vi "FuzzyMapToInt16.vi"(8 "Table Control":string[][](table)) -> (0 "Array 2":u16[](array[numeric]))   [LabVIEW 2016]
panel:
  out "Array":i32[](array[numeric])
  out "array":string[](array[string])
  out "output array":string[](array[string])
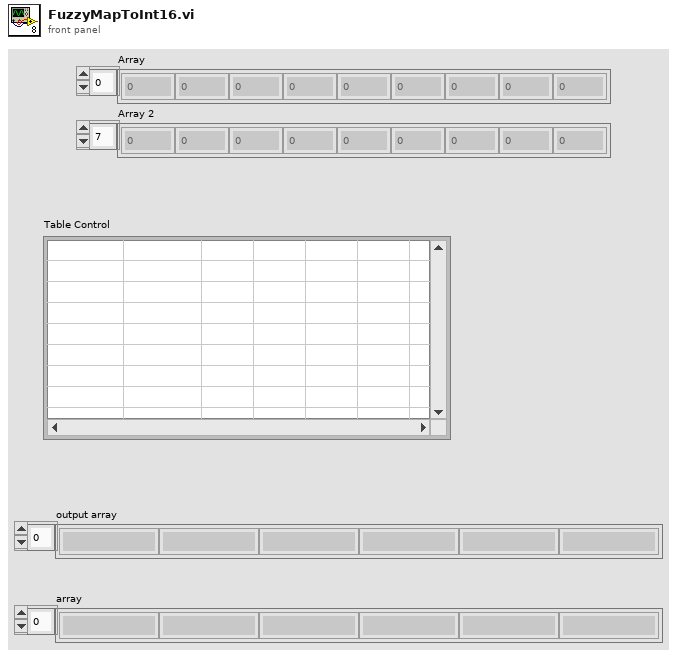
[diagram p1: front panel]
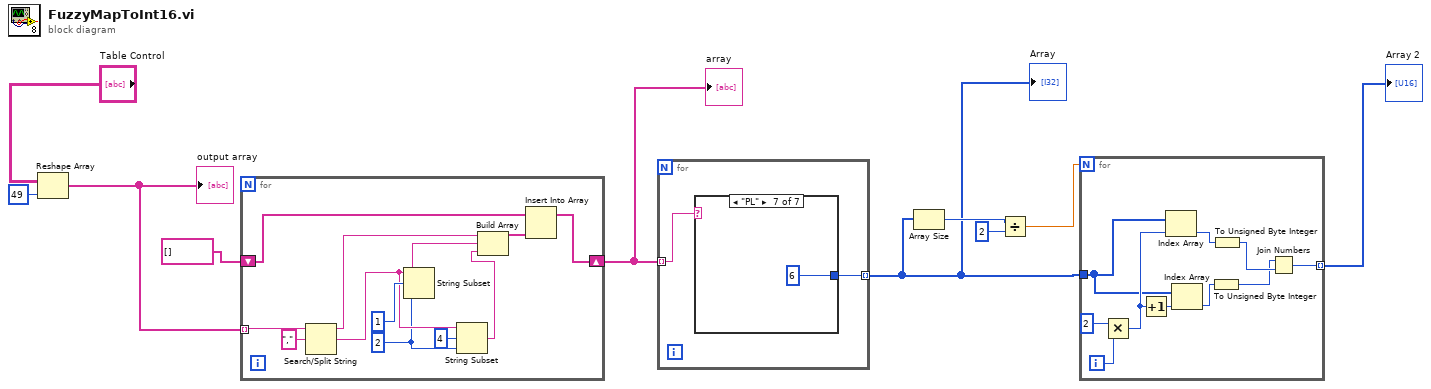
[diagram p0: block diagram]
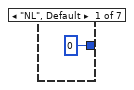
[diagram p2: hidden frame]
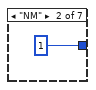
[diagram p3: hidden frame]
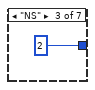
[diagram p4: hidden frame]
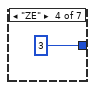
[diagram p5: hidden frame]
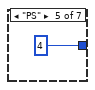
[diagram p6: hidden frame]
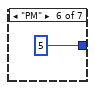
[diagram p7: hidden frame]
diagram:
  n1 = Reshape Array("Table Control", 49 ("dimension size")) -> (w8:string[])
  "output array" <- w8
  n2 = for {
    tunnel: w8 -> [w22] mode=indexing
    shift-right: [w17] -> w6
    shift-left: string[] [] ("array") -> [w18]
    w13 = 2 ("length (rest)")
    n3 = Search/Split String(string=w22, search string/char (-)=",") -> (substring before match=w20:string, match + rest of string=w14:string)  [unwired: 1 in, 1 out]
    n4 = String Subset(string=w14, offset (0)=1, length (rest)=w13) -> (substring=w15:string)
    n5 = String Subset(string=w14, offset (0)=4, length (rest)=w13) -> (substring=w11:string)
    n6 = Build Array(w20, w15, w11) -> (w19:string[])
    n7 = Insert Into Array(array=w18, new element=w19) -> (w17:string[])  [unwired: 1 in]
  }
  "array" <- w6
  n8 = for {
    tunnel: w6 -> [w24] mode=indexing
    tunnel: [w23] -> w2 mode=indexing
    n9 = case shown="\"PL\"" w24 {
      tunnel: [0 ("length (rest)") 1 ("length (rest)") 2 ("length (rest)") 3 ("length (rest)") 4 ("length (rest)") 5 ("length (rest)") 6 ("length (rest)")] -> w23
      frame "NL", Default {
      }
      frame "NM" {
      }
      frame "NS" {
      }
      frame "ZE" {
      }
      frame "PS" {
      }
      frame "PM" {
      }
      frame "PL" {
      }
    }
  }
  "Array" <- w2
  n10 = Array Size(array=w2) -> (size(s)=w5:i32)
  n11 = Divide(x=w5, y=2) -> (x/y=w3:dbl)
  n12 = for {
    N: w3 -> [_]
    tunnel: w2 -> [w37]
    tunnel: [w34] -> w1 mode=indexing
    i -> [w41]
    n13 = Multiply(x=2, y=w41) -> (x*y=w39:i32)
    n14 = Increment(x=w39) -> (x+1=w38:i32)
    n15 = Index Array(array=w37, index=w39) -> (element=w36:i32)
    n16 = Index Array(array=w37, index=w38) -> (element=w35:i32)
    n17 = To Unsigned Byte Integer(number=w35) -> (unsigned 8bit integer=w32:u8)
    n18 = To Unsigned Byte Integer(number=w36) -> (unsigned 8bit integer=w33:u8)
    n19 = Join Numbers(hi=w32, lo=w33) -> ((hi.lo)=w34:u16)
  }
  "Array 2" <- w1
